vi "Do.vi"(8 "error in (no error)":errorcluster, 10 "Actor in":refnum<class "Actor.lvclass">, 11 "Connection Msg":refnum<class "Connection Msg.lvclass">) -> (0 "error out":errorcluster, 2 "Actor out":refnum<class "Actor.lvclass">)   [LabVIEW 2025, in "PLC_Module.lvlib" / "Connection Msg.lvclass"]
doc: "This VI delivers the message to the actor by calling the appropriate method(s) on the actor."
uses:
  Connection Msg.lvclass
  <vilib>/ActorFramework/Actor/Actor.lvclass
  Connection Msg.lvclass/Connection Msg.ctl
  PLC_Module/PLC_Module.lvclass
  9ef47adc-f318-494c-9b8b-6df3216d6863.vi
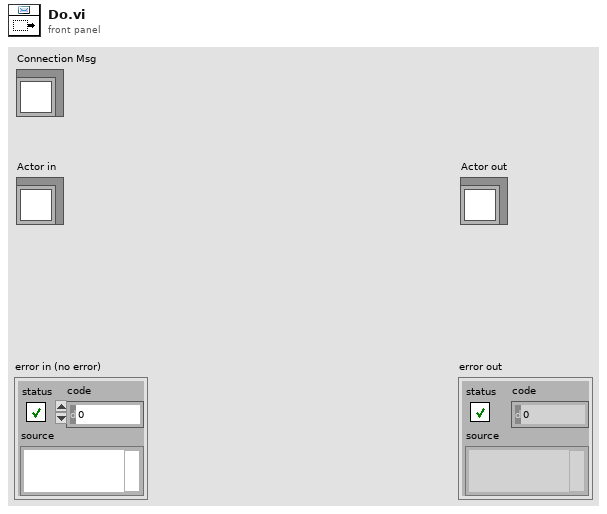
[diagram p1: front panel]
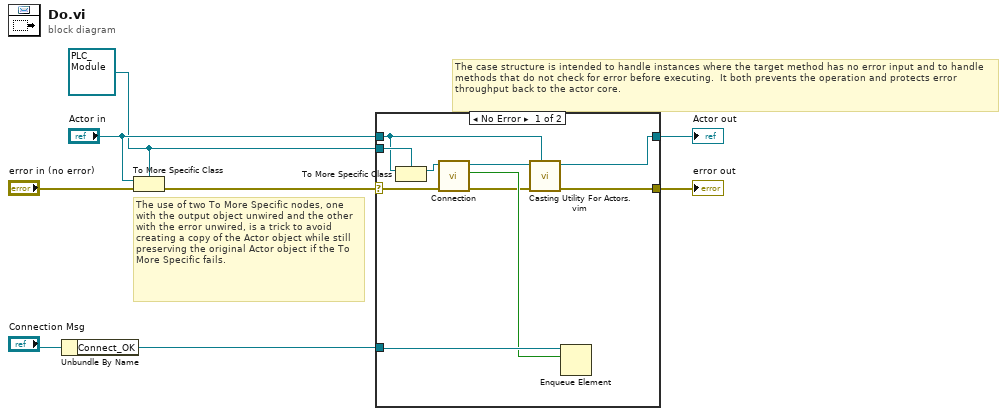
[diagram p0: block diagram]
diagram:
  w3 = refnum<class "PLC_Module.lvclass"> refnum ("Actor in")
  # "The use of two To More Specific nodes, one with the output object unwired and the other with the error unwired, is a trick to avoid creating a copy of the Actor object while still preserving the original Actor object if the To More Specific fails."
  # "The case structure is intended to handle instances where the target method has no error input and to handle methods that do not check for error before executing.  It both prevents the operation and protects error throughput back to the actor core."
  n1 = Unbundle By Name("Connection Msg") -> ("Connect_OK"=w1:refnum<queue>)
  n2 = To More Specific Class(target class=w3, reference="Actor in", error in="error in (no error)") -> (error out=w7:errorcluster)  [unwired: 1 out]
  n3 = case shown="No Error" w7 {
    selector: w7 -> [w18 w20]
    tunnel: [w12 w20] -> w6
    tunnel: [w13 w19] -> w5
    tunnel: "Actor in" -> [w15 w19]
    tunnel: w3 -> [w16 _]
    tunnel: w1 -> [w11 _]
    frame No Error {
      n4 = To More Specific Class(target class=w16, reference=w15) -> (specific class reference=w17:refnum<class "PLC_Module.lvclass">)  [unwired: 1 in, 1 out]
      n5 = call "Connection.vi"("error in (no error)"=w18, "PLC_Module in"=w17) -> ("error out"=w9:errorcluster, "Connect_OK"=w10:bool, "PLC_Module out"=w14:refnum<class "PLC_Module.lvclass">)  [unwired: 7 in]
      n6 = call "Casting Utility For Actors.vim"("type"=w15, "error in (no error)"=w9, "Actor in"=w14) -> ("error out"=w12:errorcluster, "Actor out"=w13:refnum<class "Actor.lvclass">)  [unwired: 7 in]
      n7 = Enqueue Element(queue=w11, element=w10) -> ()  [unwired: 2 in, 3 out]
    }
    frame Error {
      # "If type check fails, pass the original object out again."
    }
  }
  "error out" <- w6
  "Actor out" <- w5
